vi "ReadAttributesTest.vi"() -> ()   [LabVIEW 2013]
uses:
  <vilib>/Utility/error.llb/DialogType.ctl
  <vilib>/tango-binding-2.0.0-rc2-lv2013-windows-x64-msvc-10/vi/lv-2013/tango_vi.llb/avToDoubleScalar.vi
  <vilib>/tango-binding-2.0.0-rc2-lv2013-windows-x64-msvc-10/vi/lv-2013/tango_vi.llb/tango.lvlib
panel:
  out "value":dbl
  out "Err msg":string
  out "success":bool=TRUE
  in  "<TangoTest> device name":string="sys/tg_test/1"
  # "TANGO  Binding for LabVIEW - ReadAttributes example"
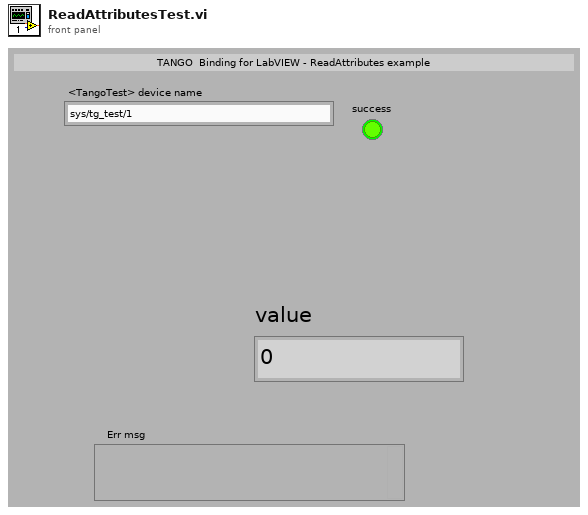
[diagram p1: front panel]
types:
  T1 = typedef "DialogType.ctl" = u16
  T2 = cluster{"device name":string, "attribute name":string, "quality value":i16, "quality string":string, "timestamp":dbl, "dim. x":i32, "dim. y":i32, "value":u8[], "error code":i32, "error stack":string[], "data type":u16}[]
  T3 = cluster{"device name":string, "attribute name":string, "quality value":i16, "quality string":string, "timestamp":dbl, "dim. x":i32, "dim. y":i32, "value":u8[], "error code":i32, "error stack":string[], "data type":u16}
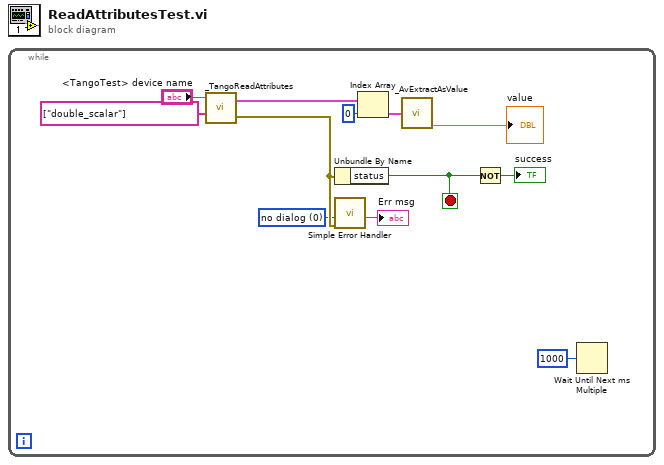
[diagram p0: block diagram]
diagram:
  n1 = while {
    stop <- w6 stop-if-true
    w3 = T1 0 items=["no dialog", "OK message", "continue or stop message", "OK message + warnings", "continue/stop + warnings"] ("type of dialog (OK msg:1)")
    n2 = call <vilib>:"_TangoReadAttributes.vi"("attribute names"=string[] ["double_scalar"], "device name"="<TangoTest> device name") -> ("error out"=w7:errorcluster, "attribute values"=w12:T2)  [unwired: 1 in]
    n3 = Unbundle By Name(w7) -> ("status"=w6:bool)
    n4 = call <vilib>:"Simple Error Handler.vi"("type of dialog (OK msg:1)"=w3, "error in (no error)"=w7) -> ("source out"=→"Err msg":string)  [unwired: 3 in, 4 out]
    n5 = Index Array(array=w12, index=0 ("indice")) -> (element=w9:T3)
    n6 = call-poly <vilib>:"_AvExtractAsValue.vi"("attribute value"=w9) -> ("value"=→"value":dbl)  [unwired: 4 out]
    n7 = Not(x=w6) -> (.not. x?=→"success":bool)
    n8 = Wait Until Next ms Multiple(millisecond multiple=u32 1000) -> ()  [unwired: 1 out]
  }
